vi "pixel pulse gen.vi"(2 "error in":errorcluster, 3 "Y line":i32=400, 4 "X pixel":i32=400) -> (0 "error out":errorcluster, 1 "digital waveform out":digitalwaveform(waveform)={"t0"=timestamp(0 s since 1904-01-01), "dt"=1.0, "Y"={"transitions"=[], "data"=[]}})   [LabVIEW 2012]
uses:
  <vilib>/Waveform/DWDTOps.llb/Digital Pattern Generator (Toggle).vi
  <vilib>/Waveform/DWDTOps.llb/Digital Pattern Generator (Single Value).vi
  <vilib>/Waveform/DWDTOps.llb/DWDT Append Digital Samples.vi
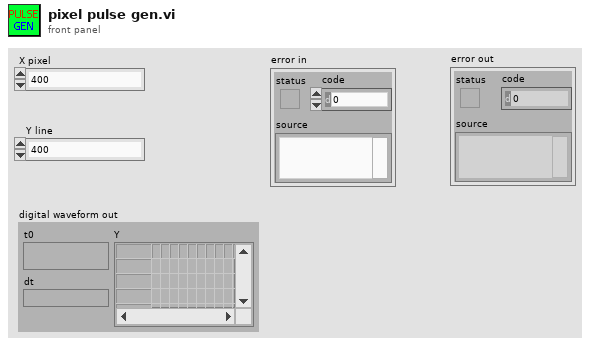
[diagram p1: front panel]
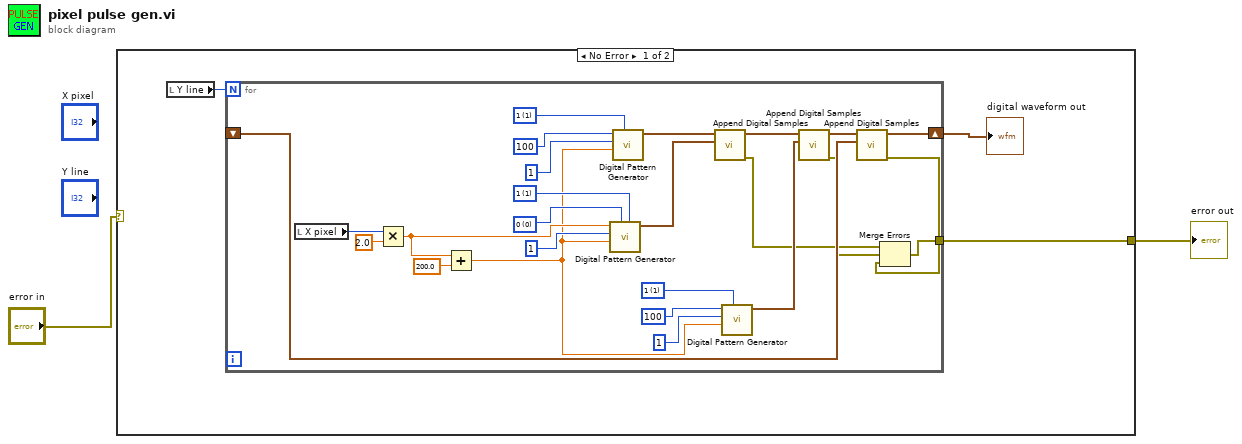
[diagram p0: block diagram]
diagram:
  n1 = case shown="No Error" "error in" {
    selector: "error in" -> [_ w31]
    tunnel: [w3 w31] -> w1
    frame No Error {
      n2 = local read "Y line"() -> (w5:i32)
      n3 = for {
        N: w5 -> [_]
        shift-right: [w17] -> w4
        shift-left: _ -> [w15]
        tunnel: [w6] -> w3
        w22 = u8 1 items=["0", "1", "Z", "L", "H", "X", "T", "V"] ("value 2")
        w24 = u8 0 items=["0", "1", "Z", "L", "H", "X", "T", "V"] ("value")
        w27 = u8 1 items=["0", "1", "Z", "L", "H", "X", "T", "V"] ("value")
        w30 = u8 1 items=["0", "1", "Z", "L", "H", "X", "T", "V"] ("value")
        n4 = local read "X pixel"() -> (w13:i32)
        n5 = Multiply(x=w13, y=2.0) -> (x*y=w11:dbl)
        n6 = Add(x=w11, y=200.0) -> (x+y=w10:dbl)
        n7 = call-poly <vilib>:"Digital Pattern Generator.vi"("value 2"=w22, "value 1"=w24, "sample rate"=w10, "number of signals"=u32 1, "number of samples"=w11) -> ("digital waveform"=w20:digitalwaveform)  [unwired: 1 in, 5 out]
        n8 = call-poly <vilib>:"Digital Pattern Generator.vi"("value"=w30, "sample rate"=w10, "number of signals"=u32 1, "number of samples"=u32 100) -> ("digital waveform"=w21:digitalwaveform)  [unwired: 1 in, 6 out]
        n9 = call-poly <vilib>:"Append Digital Samples.vi"("digital waveform B"=w20, "digital waveform A"=w21) -> ("error out"=w9:errorcluster, "digital waveform out"=w19:digitalwaveform)  [unwired: 1 in, 7 out]
        n10 = call-poly <vilib>:"Digital Pattern Generator.vi"("value"=w27, "sample rate"=w10, "number of signals"=u32 1, "number of samples"=u32 100) -> ("digital waveform"=w18:digitalwaveform)  [unwired: 1 in, 6 out]
        n11 = call-poly <vilib>:"Append Digital Samples.vi"("digital waveform B"=w18, "digital waveform A"=w19) -> ("error out"=w8:errorcluster, "digital waveform out"=w16:digitalwaveform)  [unwired: 1 in, 7 out]
        n12 = call-poly <vilib>:"Append Digital Samples.vi"("digital waveform B"=w15, "digital waveform A"=w16) -> ("error out"=w7:errorcluster, "digital waveform out"=w17:digitalwaveform)  [unwired: 1 in, 7 out]
        n13 = Merge Errors(w9, w8, w7) -> (w6:errorcluster)
      }
      "digital waveform out" <- w4
    }
    frame Error {
    }
  }
  "error out" <- w1
